vi "test_fit_SOS.vi"() -> ()   [LabVIEW 2017]
uses:
  controls/SOS_frf_data.ctl
  controls/fit_sos_results.ctl
  controls/FrdData.ctl
  <vilib>/addons/_JKI.lib/Serialization/JSON/JKI JSON Serialization.lvlib
panel:
  out "K":dbl
  out "Den":dbl[](array[numeric])
  out "Num":dbl[](array[numeric])
  out "FRD-array":T1[](array[typedef])
  out "theta0":dbl[](array[numeric])
  out "Bode amplitude 2":cluster{"W":dbl[], "Magnitude":dbl[]}[](graph) caption="Magnitude Graph"
  out "error out":errorcluster
  out "fit_sos_result":T2
  out "SOS-frf_data":T3
  in  "error in (no error)":errorcluster
  in  "system data path":path=path "C:/Users/arnold/Documents/afm-cs/c-src/frf_test_data.json"
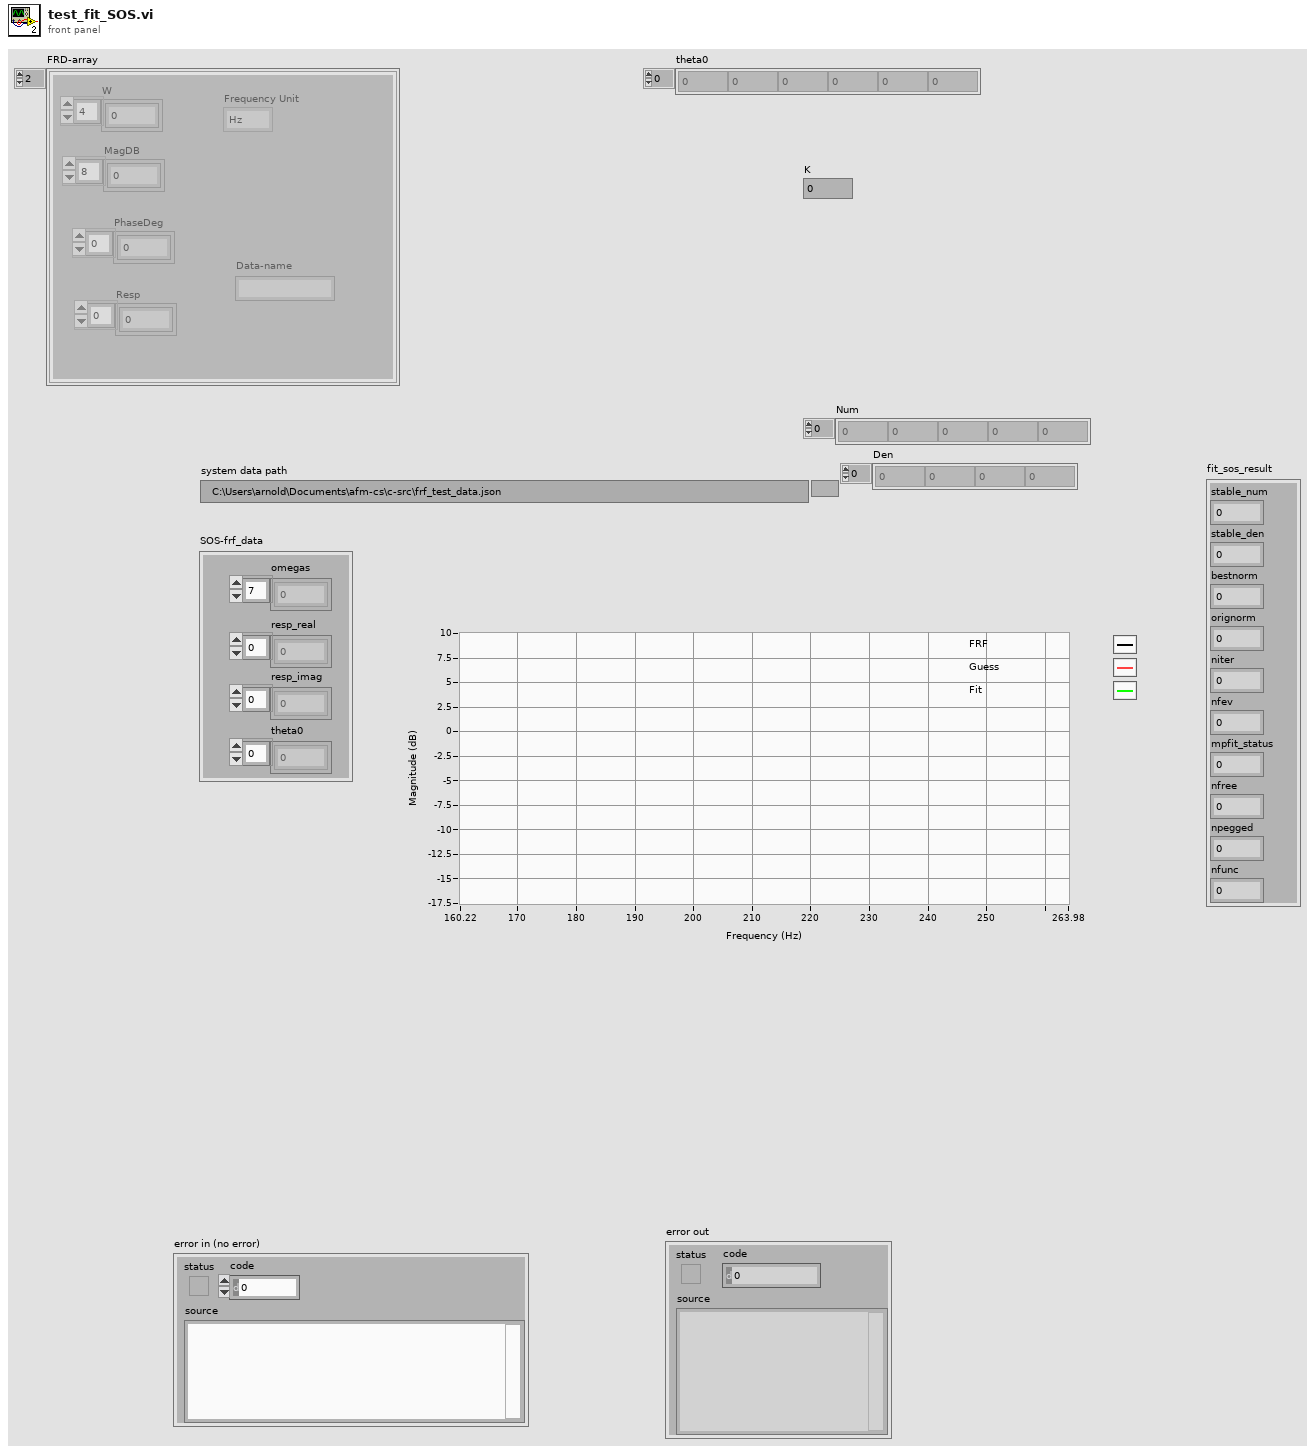
[diagram p1: front panel]
types:
  T1 = typedef "FrdData.ctl" = cluster{"Frequency Unit":enum16{"Hz", "rad/s"}, "W":dbl[], "MagDB":dbl[], "PhaseDeg":dbl[], "Resp":cdb[], "Data-name":string}
  T2 = typedef "fit_sos_results.ctl" = cluster{"stable_num":i32, "stable_den":i32, "bestnorm":dbl, "orignorm":dbl, "niter":i32, "nfev":i32, "mpfit_status":i32, "nfree":i32, "npegged":i32, "nfunc":i32}
  T3 = typedef "SOS_frf_data.ctl" = cluster{"omegas":dbl[], "resp_real":dbl[], "resp_imag":dbl[], "theta0":dbl[]}
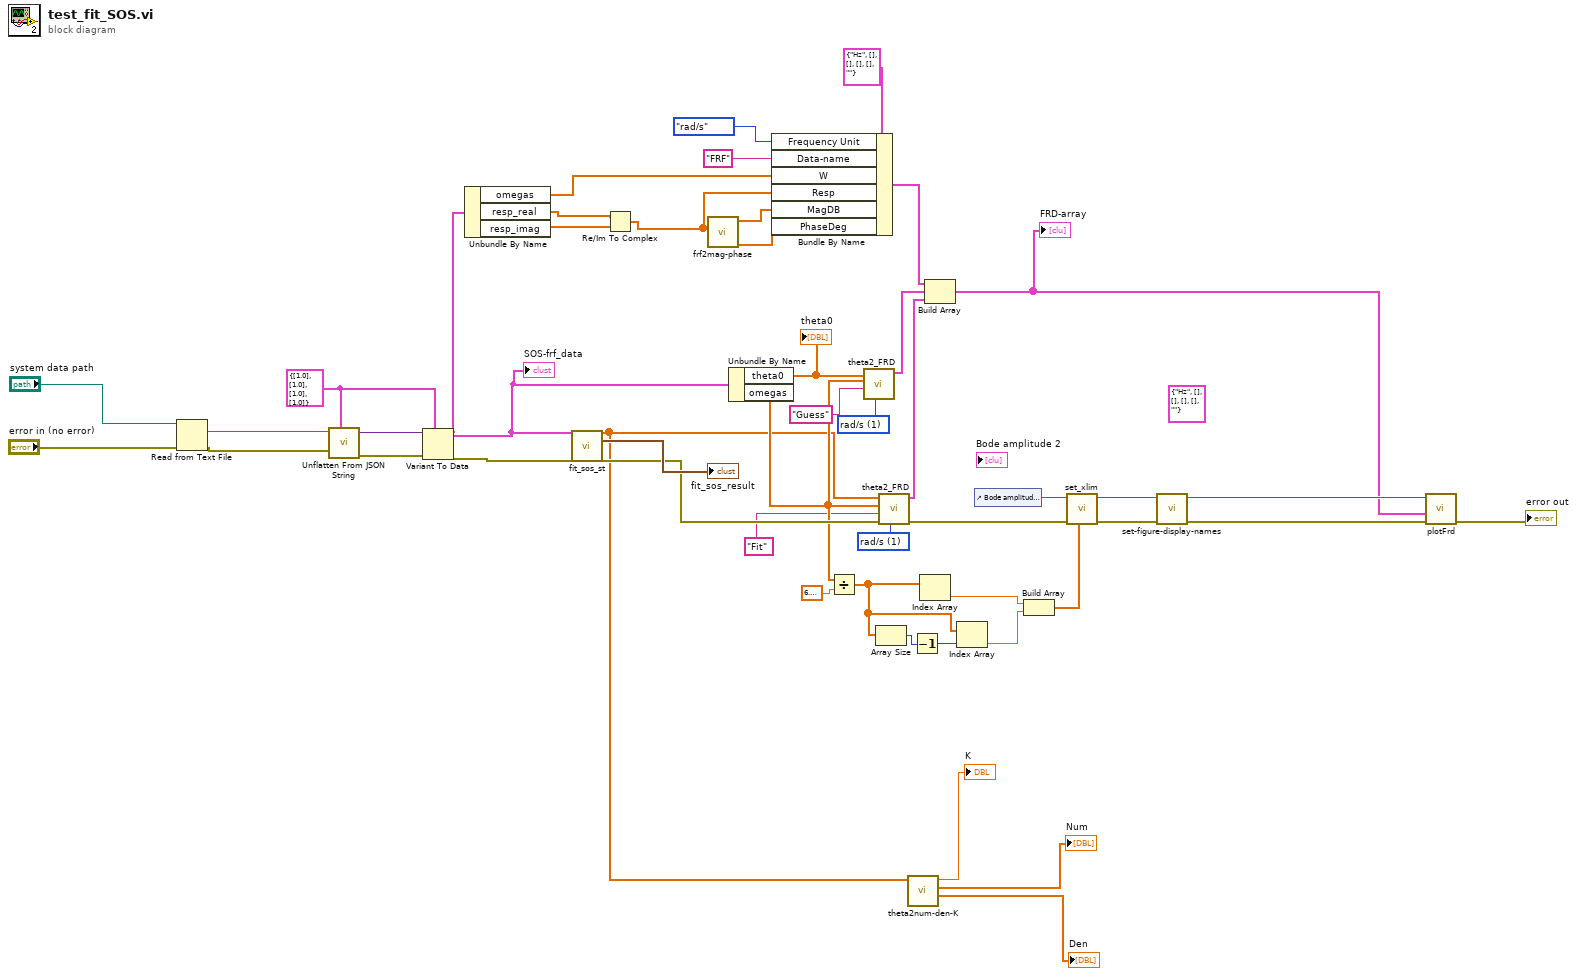
[diagram p0: block diagram]
diagram:
  (unwired) T1 {"Frequency Unit"=enum."Hz", "W"=[], "MagDB"=[], "PhaseDeg"=[], "Resp"=[], "Data-name"=""} ("FrdData Out 2")
  w16 = u16 1 items=["Hz", "rad/s"] ("freq unit")
  w17 = u16 1 items=["Hz", "rad/s"] ("freq unit")
  w40 = T3 {"omegas"=[1.0], "resp_real"=[1.0], "resp_imag"=[1.0], "theta0"=[1.0]} ("frf_data")
  n1 = Read from Text File(file (use dialog)="system data path", error in="error in (no error)") -> (text=w46:string, error out=w45:errorcluster)  [unwired: 2 in, 2 out]
  n2 = call <vilib>:"Unflatten From JSON String.vi"("Type and Defaults"=w40, "error in (no error)"=w45, "JSON String"=w46) -> ("error out"=w47:errorcluster, "Variant"=w48:variant)  [unwired: 7 in]
  n3 = Variant To Data(error in=w47, type=w40, Variant=w48) -> (data=w35:T3, error out=w42:errorcluster)
  "SOS-frf_data" <- w35
  n4 = Unbundle By Name(w35) -> ("omegas"=w11:dbl[], "resp_real"=w38:dbl[], "resp_imag"=w37:dbl[])
  n5 = call "fit_sos_st.vi"("frf_data"=w35, "error in (no error)"=w42) -> ("theta"=w4:dbl[], "fit_sos_result"=→"fit_sos_result":T2, "error out"=w39:errorcluster)  [unwired: 23 in]
  n6 = Re/Im To Complex(1:w37, 2:w38) -> (0:w12:cdb[])
  n7 = call "frf2mag-phase.vi"("G_frf"=w12) -> ("phase [deg]"=w14:dbl[], "mag-dB"=w13:dbl[])  [unwired: 9 in]
  n8 = Unbundle By Name(w35) -> ("theta0"=w18:dbl[], "omegas"=w19:dbl[])
  "theta0" <- w18
  n9 = Bundle By Name(cluster=T1 {"Frequency Unit"=enum."Hz", "W"=[], "MagDB"=[], "PhaseDeg"=[], "Resp"=[], "Data-name"=""} ("FRD-model"), "Frequency Unit"=enum16{"Hz", "rad/s"}."rad/s", "Data-name"="FRF" ("Data_name"), "W"=w11, "Resp"=w12, "MagDB"=w13, "PhaseDeg"=w14) -> (w7:T1)
  n10 = Divide(x=w19, y=6.283185307179586) -> (x/y=w24:dbl[])
  n11 = call "theta2_FRD.vi"("freq unit"=w17, "Data-name"="Guess", "freqs/omega"=w19, "theta"=w18) -> ("FRD-model"=w20:T1)  [unwired: 6 in, 1 out]
  n12 = Array Size(array=w24) -> (size(s)=w22:i32)
  n13 = call "theta2_FRD.vi"("freq unit"=w16, "error in (no error)"=w39, "Data-name"="Fit", "freqs/omega"=w19, "theta"=w4) -> ("error out"=w33:errorcluster, "FRD-model"=w21:T1)  [unwired: 5 in]
  n14 = call "theta2num-den-K.vi"("theta"=w4) -> ("Den"=→"Den":dbl[], "Num"=→"Num":dbl[], "K"=→"K":dbl)  [unwired: 8 in]
  n15 = Decrement(x=w22) -> (x-1=w23:i32)
  n16 = Index Array(array=w24) -> (element=w27:dbl)  [unwired: 1 in]
  n17 = Build Array(w7, w20, w21) -> (w6:T1[])
  "FRD-array" <- w6
  n18 = Index Array(array=w24, index=w23) -> (element=w28:dbl)
  n19 = control-ref of="Bode amplitude 2"() -> (w34:refnum<vi>)
  n20 = Build Array(w27, w28) -> (w26:dbl[])
  n21 = call "set_xlim.vi"("xlim"=w26, "error in"=w33, "figure (in)"=w34) -> ("error out"=w32:errorcluster, "figure (out)"=w29:refnum<vi>)  [unwired: 7 in]
  n22 = call "set-figure-display-names.vi"("error in"=w32, "figure (in)"=w29) -> ("error out"=w31:errorcluster, "figure (out)"=w30:refnum<vi>)  [unwired: 8 in]
  n23 = call "plotFrd.vi"("error in (no error)"=w31, "FRD-array"=w6, "Magnitude Graph Reference in"=w30) -> ("error out"=→"error out":errorcluster)  [unwired: 6 in, 2 out]
